vi "Reshaper1.vi"(3 "error IN":errorcluster, 5 "[IN] (X,Y,dX,dY)":dbl[][](array[numeric])) -> (0 "error OUT":errorcluster, 1 "Numeric":i32, 2 "[OUT] Reshaped (X,Y,dX,dY)":dbl[][](array[numeric]))   [LabVIEW 2013]
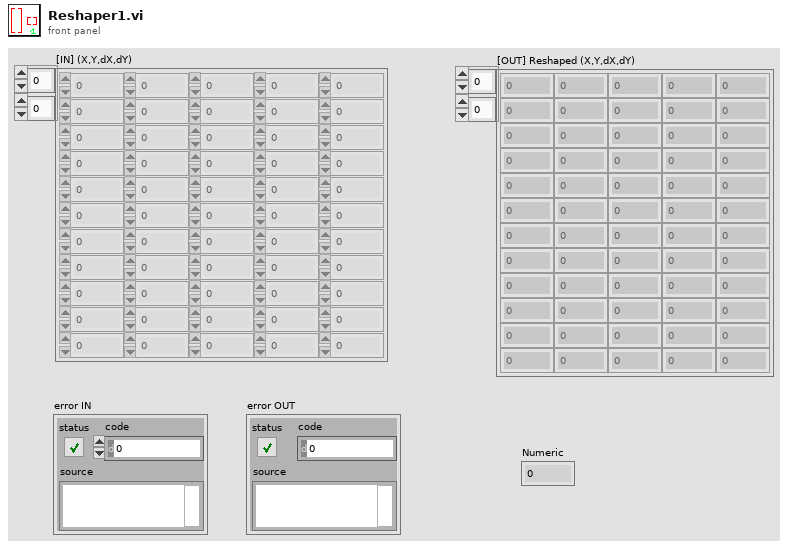
[diagram p1: front panel]
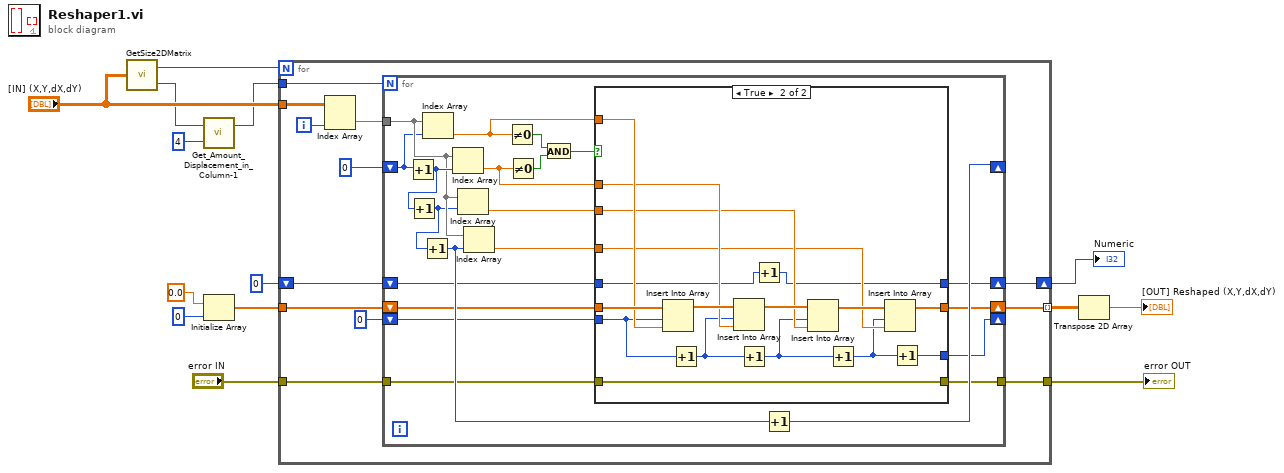
[diagram p0: block diagram]
diagram:
  n1 = call "GetSize2DMatrix.vi"("Array IN (2D)"="[IN] (X,Y,dX,dY)") -> ("# Cols"=w4:i32, "# Rows"=w3:i32)
  n2 = call "Get_Amount_Displacement_in_Column-1.vi"("multiplier"=4, "# Rows"=w3) -> ("Displ amount"=w1:i32)  [unwired: 1 out]
  n3 = Initialize Array(0.0 ("element"), 0 ("dimension size")) -> (w12:dbl[])
  n4 = for {
    N: w4 -> [_]
    tunnel: "[IN] (X,Y,dX,dY)" -> [w26]
    tunnel: w12 -> [w22]
    tunnel: [w21] -> w11 mode=indexing
    tunnel: "error IN" -> [w20]
    tunnel: [w19] -> w8
    shift-right: [w17] -> w6
    shift-left: 0 -> [w18]
    tunnel: w1 -> [w15]
    i -> [w25]
    n5 = Index Array(array=w26, index (col)=w25) -> (element=w24:dbl[])  [unwired: 1 in]
    n6 = for {
      N: w15 -> [_]
      tunnel: w24 -> [w46]
      shift-right: [w41] -> _
      shift-left: 0 -> [w38]
      shift-right: [w33] -> w21
      shift-left: w22 -> [w39]
      tunnel: w20 -> [w32]
      tunnel: [w31] -> w19
      shift-right: [w29] -> w17
      shift-left: w18 -> [w30]
      shift-right: [w27] -> _
      shift-left: 0 -> [w28]
      n7 = Increment(x=w38) -> (x+1=w47:i32)
      n8 = Increment(x=w47) -> (x+1=w45:i32)
      n9 = Increment(x=w45) -> (x+1=w42:i32)
      n10 = Index Array(array=w46, index=w38) -> (element=w37:dbl)
      n11 = Index Array(array=w46, index=w47) -> (element=w36:dbl)
      n12 = Index Array(array=w46, index=w45) -> (element=w35:dbl)
      n13 = Index Array(array=w46, index=w42) -> (element=w34:dbl)
      n14 = Not Equal To 0?(x=w37) -> (x != 0?=w43:bool)
      n15 = Not Equal To 0?(x=w36) -> (x != 0?=w44:bool)
      n16 = And(x=w43, y=w44) -> (x .and. y?=w40:bool)
      n17 = case shown="True" w40 {
        tunnel: w39 -> [w51 w68]
        tunnel: w28 -> [w48 w66]
        tunnel: w37 -> [_ w67]
        tunnel: w36 -> [_ w64]
        tunnel: w35 -> [_ w62]
        tunnel: w34 -> [_ w59]
        tunnel: [w51 w57] -> w33
        tunnel: w32 -> [w50 w56]
        tunnel: [w50 w56] -> w31
        tunnel: w30 -> [w49 w55]
        tunnel: [w49 w54] -> w29
        tunnel: [w48 w52] -> w27
        frame False {
        }
        frame True {
          n18 = Insert Into Array(array=w68, index=w66, new element=w67) -> (w65:dbl[])
          n19 = Increment(x=w66) -> (x+1=w61:i32)
          n20 = Insert Into Array(array=w65, index=w61, new element=w64) -> (w63:dbl[])
          n21 = Increment(x=w61) -> (x+1=w58:i32)
          n22 = Increment(x=w55) -> (x+1=w54:i32)
          n23 = Insert Into Array(array=w63, index=w58, new element=w62) -> (w60:dbl[])
          n24 = Increment(x=w58) -> (x+1=w53:i32)
          n25 = Insert Into Array(array=w60, index=w53, new element=w59) -> (w57:dbl[])
          n26 = Increment(x=w53) -> (x+1=w52:i32)
        }
      }
      n27 = Increment(x=w42) -> (x+1=w41:i32)
    }
  }
  "error OUT" <- w8
  "Numeric" <- w6
  n28 = Transpose 2D Array(2D array=w11) -> (transposed array=→"[OUT] Reshaped (X,Y,dX,dY)":dbl[][])
